vi "Perform Radio Test.vi"(8 "error in (no error)":errorcluster, 11 "LCM Single-Up MTS Test in":refnum<class "LCM Single-Up MTS Test.lvclass">) -> (0 "error out":errorcluster, 3 "Radio Test Passed":bool)   [LabVIEW 2015, in "LCM Single-Up MTS Test.lvclass"]
uses:
  LCM Single-Up MTS Test.lvclass
  <vilib>/Cree, Inc/Cree Test Framework/Core Launcher/Core Manager Methods -- Enum.ctl
  <vilib>/Cree, Inc/Cree Test Framework/Classes/Base Objects/Base Class/Base Class/Base Class.lvclass
  <vilib>/Cree, Inc/Cree Test Framework/Core Launcher/Core Launcher.lvlib
  <vilib>/Cree, Inc/Cree Test Framework/Classes/Data/Data Repo/Class/Data Repo.lvclass
  Classes/Manufacturing Test/Class/SC Manufacturing Test.lvclass
  Classes/Test Recipe/Class/Test Recipe.lvclass
  Classes/Application/Class/Application.lvclass
  Test Class/Test Class.lvclass
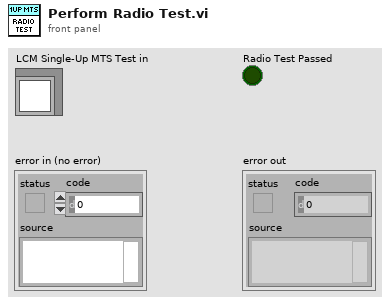
[diagram p1: front panel]
types:
  T1 = typedef "Core Launcher.lvlib/Core Manager Methods -- Enum.ctl" = enum16{"Spawn Objects", "Get Objects", "Destroy Objects"}
  T2 = typedef "Application.lvlib/App Properties.lvclass/Class Properties -- Cluster.ctl" = cluster{"UUT Info":T3[], "Test Information":refnum<vi>, "Test Complete Event":refnum<user-event>, "Shop Floor System":refnum<class "Shop Floor System.lvclass">, "Gold Board":refnum<class "Golden Board.lvclass">, "Test Recipe":refnum<class "Test Recipe.lvclass">, "Instruments":refnum<class "Instrument.lvclass">[], "Mode":T4, "Test Results":cluster{"Pass":bool[], "Fail Codes":string[]}, "Station Config":refnum<class "Station Config.lvclass">}
  T3 = typedef "Application.lvlib/App Properties.lvclass/UUT Reference -- Cluster.ctl" = cluster{"Serial Number Reference":refnum<vi>, "Status Message Reference":refnum<vi>}
  T4 = typedef "Application.lvlib/Application.lvclass/Op Mode -- Enum.ctl" = u16
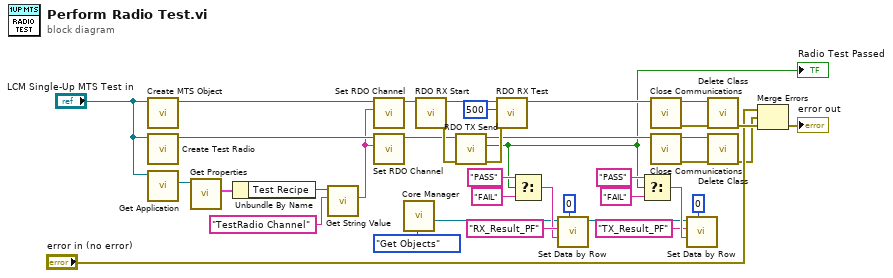
[diagram p0: block diagram]
diagram:
  n1 = call "Create MTS Object.vi"("LCM Single-Up MTS Test in"="LCM Single-Up MTS Test in") -> ("MTS"=w21:refnum<class "SC Manufacturing Test.lvclass">)  [unwired: 9 in, 1 out]
  n2 = call "Create Test Radio.vi"("LCM Single-Up MTS Test in"="LCM Single-Up MTS Test in") -> ("Test Radio"=w20:refnum<class "SC Manufacturing Test.lvclass">)  [unwired: 9 in, 1 out]
  n3 = call "Get Application.vi"("Test Class in"="LCM Single-Up MTS Test in") -> ("Application.lvlib:Application.lvclass"=w18:refnum<class "Application.lvclass">)  [unwired: 9 in, 1 out]
  n4 = call "Get Properties.vi"("Acrobat Template in"=w18) -> ("Class Properties"=w17:T2)  [unwired: 8 in, 2 out]
  n5 = Unbundle By Name(w17) -> ("Test Recipe"=w19:refnum<class "Test Recipe.lvclass">)
  n6 = call "Get String Value.vi"("Name"="TestRadio Channel", "Test Recipe in"=w19) -> ("Value"=w15:string)  [unwired: 7 in, 2 out]
  n7 = call "Set RDO Channel.vi"("Channel"=w15, "Acrobat Template in"=w21) -> ("Acrobat Template out"=w8:refnum<class "SC Manufacturing Test.lvclass">)  [unwired: 8 in, 1 out]
  n8 = call "Set RDO Channel.vi"("Channel"=w15, "Acrobat Template in"=w20) -> ("Acrobat Template out"=w9:refnum<class "SC Manufacturing Test.lvclass">)  [unwired: 8 in, 1 out]
  n9 = call <vilib>:"Core Manager.vi"("Method"=Core_Manager_Methods_--_Enum."Get Objects") -> ("Data Repo"=w23:refnum<class "Data Repo.lvclass">)  [unwired: 7 in, 3 out]
  n10 = call "RDO RX Start.vi"("Acrobat Template in"=w8) -> ("error out"=w11:errorcluster, "Acrobat Template out"=w13:refnum<class "SC Manufacturing Test.lvclass">)  [unwired: 9 in]
  n11 = call "RDO TX Send.vi"("error in (no error)"=w11, "Acrobat Template in"=w9) -> ("error out"=w12:errorcluster, "Passed"=w1:bool, "Acrobat Template out"=w5:refnum<class "SC Manufacturing Test.lvclass">)  [unwired: 7 in]
  "Radio Test Passed" <- w1
  n12 = call "RDO RX Test.vi"("error in (no error)"=w12, "Time to Wait (2000 ms)"=u32 500, "Acrobat Template in"=w13) -> ("Acrobat Template out"=w4:refnum<class "SC Manufacturing Test.lvclass">)  [unwired: 5 in, 3 out]
  n13 = Select(t="PASS" ("Header"), s=w1, f="FAIL" ("Header")) -> (s? t:f=w25:string)
  n14 = call <vilib>:"Set Data by Row.vi"("Row"=0, "Value"=w25, "Header"="RX_Result_PF", "Acrobat Template in"=w23) -> ("Acrobat Template out"=w22:refnum<class "Data Repo.lvclass">)  [unwired: 6 in, 1 out]
  n15 = Select(t="PASS" ("Header"), s=w1, f="FAIL" ("Header")) -> (s? t:f=w36:string)
  n16 = call "Close Communications.vi"("Acrobat Template in"=w4) -> ("error out"=w30:errorcluster, "Acrobat Template out"=w29:refnum<class "SC Manufacturing Test.lvclass">)  [unwired: 9 in]
  n17 = call "Close Communications.vi"("Acrobat Template in"=w5) -> ("error out"=w6:errorcluster, "Acrobat Template out"=w7:refnum<class "SC Manufacturing Test.lvclass">)  [unwired: 9 in]
  n18 = call <vilib>:"Set Data by Row.vi"("Row"=0, "Value"=w36, "Header"="TX_Result_PF", "Acrobat Template in"=w22) -> ()  [unwired: 6 in, 2 out]
  n19 = call <vilib>:"Delete Class.vi"("error in (no error)"=w30, "Base Class in"=w29) -> ("error out"=w32:errorcluster)  [unwired: 8 in, 1 out]
  n20 = call <vilib>:"Delete Class.vi"("error in (no error)"=w6, "Base Class in"=w7) -> ("error out"=w2:errorcluster)  [unwired: 8 in, 1 out]
  n21 = Merge Errors("error in (no error)", w2, w32) -> (→"error out":errorcluster)
